vi "Check all exhausted.vi"(8 "error in (no error)":errorcluster, 11 "Pool":T1[](array[typedef])=[{"index"=0, "state"=enum."unused"}, {"index"=1, "state"=enum."unused"}, {"index"=2, "state"=enum."unused"}, {"index"=3, "state"=enum."unused"}, {"index"=4, "state"=enum."unused"}, {"index"=5, "state"=enum."unused"}]) -> (0 "error out":errorcluster, 3 "T = all items are \"exhausted\"":bool)   [LabVIEW 2021, in "Numeric Utilities.lvlib"]
uses:
  Numeric Utilities.lvlib
  cluster-touched index.ctl
  index state enum.ctl
panel:
  out "Loop iteration":i32
  # "Development\ncontrols/indicators useful for development and testing, but which are not outputs of the VI"
  # "Input\nInputs to the VI"
  # "Output\nOutputs of the VI"
  # "Description\n\nBlank VI with error handling case. \n\nSummarize the use of this VI in this space."
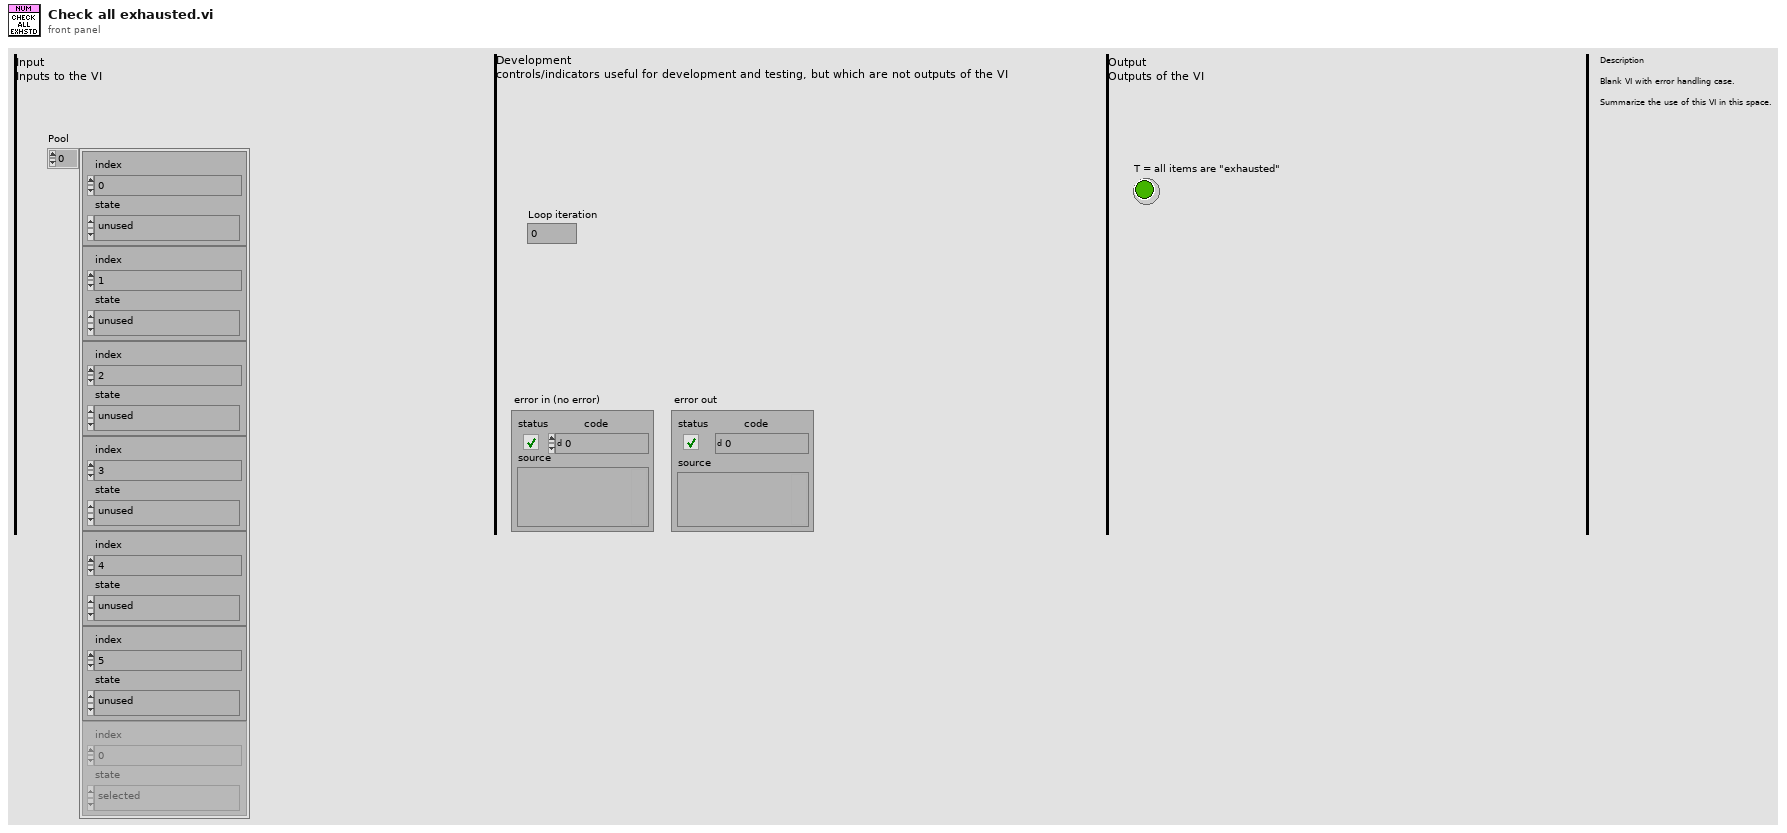
[diagram p1: front panel]
types:
  T1 = typedef "Numeric Utilities.lvlib/cluster-touched index.ctl" = cluster{"index":i32, "state":T2}
  T2 = typedef "Numeric Utilities.lvlib/index state enum.ctl" = enum16{"unused", "selected", "exhausted"}
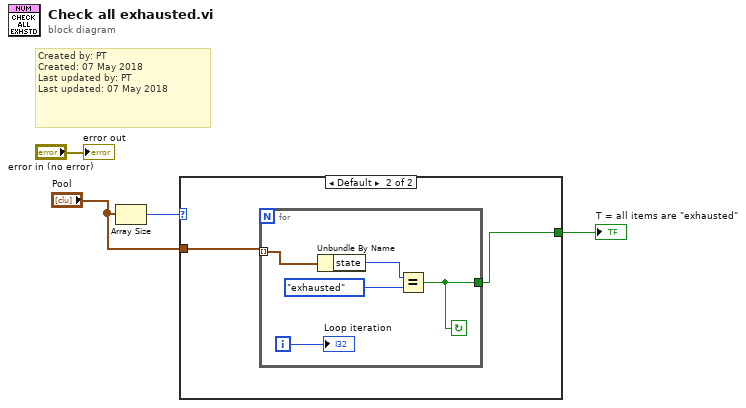
[diagram p0: block diagram]
diagram:
  # "Created by: PT\nCreated: 07 May 2018\nLast updated by: PT\nLast updated: 07 May 2018"
  n1 = Array Size(array="Pool") -> (size(s)=w2:i32)
  n2 = case shown="Default" w2 {
    tunnel: "Pool" -> [_ w6]
    tunnel: [_ w5] -> w1
    frame 0 {
    }
    frame Default {
      n3 = for {
        tunnel: w6 -> [w9] mode=indexing
        tunnel: [w8] -> w5
        i -> [w7]
        stop <- w8 continue-if-true
        n4 = Unbundle By Name(w9) -> ("state"=w11:T2)
        n5 = Equal?(x=w11, y=index_state_enum."exhausted") -> (x = y?=w8:bool)
        "Loop iteration" <- w7
      }
    }
  }
  "T = all items are \"exhausted\"" <- w1
  "error out" <- "error in (no error)"
